vi "Setup.vi"(10 "Setup":T1, 11 "Core Actor in":refnum<class "Core Actor.lvclass">) -> (0 "Error out":errorcluster, 3 "Core Actor out":refnum<class "Core Actor.lvclass">)   [LabVIEW 2025, in "jettl.lvlib" / "Actor.lvlib" / "Core Actor.lvclass"]
uses:
  Core Actor.lvclass
  Setup.ctl
  Attributes/Attributes/Attributes.lvclass
  Msg Set.ctl
  Msg/Msg.lvclass
  Attributes.ctl
  Core Actor.lvclass/Core Actor.ctl
  Attributes/Attributes.lvlib
  Actor.lvlib
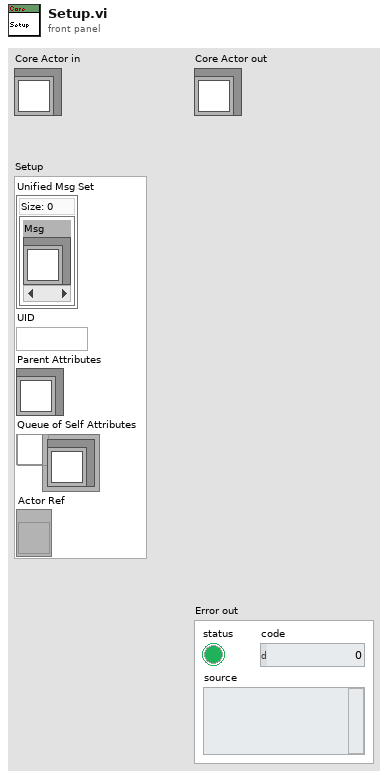
[diagram p1: front panel]
types:
  T1 = typedef "jettl.lvlib/Actor.lvlib/Setup.ctl" = cluster{"Unified Msg Set":T2, "UID":string, "Parent Attributes":refnum<class "Attributes.lvclass">, "Queue of Self Attributes":refnum<queue>, "Actor Ref":refnum<vi>}
  T2 = typedef "jettl.lvlib/Actor.lvlib/Msg Set.ctl" = set{refnum<class "Msg.lvclass">}
  T3 = typedef "jettl.lvlib/Actor.lvlib/Attributes.ctl" = cluster{"UID":string, "Address":refnum<user-event>, "Event Ref":refnum<event-registration>, "Unified Msg Set":T2, "Actor Ref":refnum<vi>, "Application Ref":refnum<vi>}
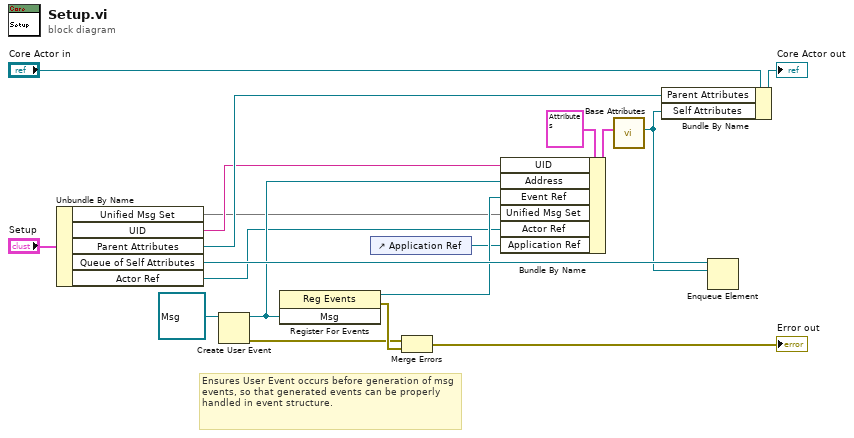
[diagram p0: block diagram]
diagram:
  # "Ensures User Event occurs before generation of msg events, so that generated events can be properly handled in event structure."
  n1 = Unbundle By Name("Setup") -> ("Unified Msg Set"=w4:T2, "UID"=w7:string, "Parent Attributes"=w10:refnum<class "Attributes.lvclass">, "Queue of Self Attributes"=w11:refnum<queue>, "Actor Ref"=w3:refnum<vi>)
  n2 = Create User Event(user event datatype=refnum<class "Msg.lvclass"> refnum ("Msg")) -> (user event=w6:refnum<user-event>, error out=w17:errorcluster)  [unwired: 1 in]
  n3 = register-events(w6) -> (reference out=w5:refnum<event-registration>, error out=w18:errorcluster)  [unwired: 2 in]
  n4 = control-ref of="Application Ref"() -> (w2:refnum<vi>)
  n5 = Merge Errors(w17, w18) -> (→"Error out":errorcluster)
  n6 = Bundle By Name(cluster=T3 {"UID"="", "Address"=refnum, "Event Ref"=refnum, "Unified Msg Set"={}, "Actor Ref"=refnum, "Application Ref"=refnum} ("Attributes"), "UID"=w7, "Address"=w6, "Event Ref"=w5, "Unified Msg Set"=w4, "Actor Ref"=w3, "Application Ref"=w2) -> (w1:T3)
  n7 = call "Base Attributes.vi"("Attributes"=w1) -> ("Attributes"=w9:refnum<class "Attributes.lvclass">)  [unwired: 10 in]
  n8 = Bundle By Name(cluster="Core Actor in", "Parent Attributes"=w10, "Self Attributes"=w9) -> (→"Core Actor out":refnum<class "Core Actor.lvclass">)
  n9 = Enqueue Element(queue=w11, element=w9) -> ()  [unwired: 2 in, 3 out]
